vi "GlobalVariables.vi"() -> ()   [LabVIEW 2014]
panel:
  out "32bit Integer Array":i32[](array[numeric])
  in  "32bit Integer":i32
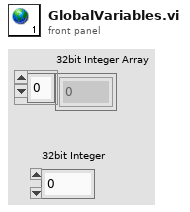
[diagram p1: front panel]
diagram:
